vi "_GetBitfiledValue.vi"(8 "error in":errorcluster, 10 "bitfield caps":T1={"offset"=0, "size"=0, "signed?"=TRUE}, 11 "register value":u64=9199446298756579247 format="%.0x") -> (0 "error out":errorcluster, 3 "bitfield balue":variant)   [LabVIEW 2017, in "Bitfield.lvlib"]
uses:
  Bitfield.lvlib
  BitfieldCaps.ctl
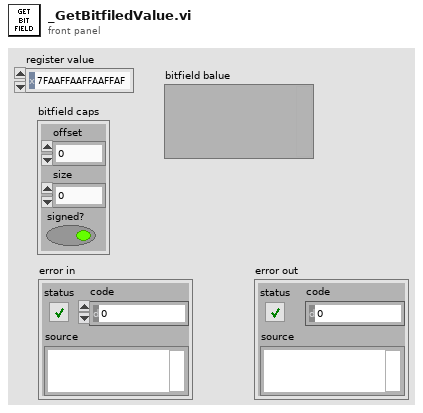
[diagram p1: front panel]
types:
  T1 = typedef "Bitfield.lvlib/BitfieldCaps.ctl" = cluster{"offset":i32, "size":i32, "signed?":bool}
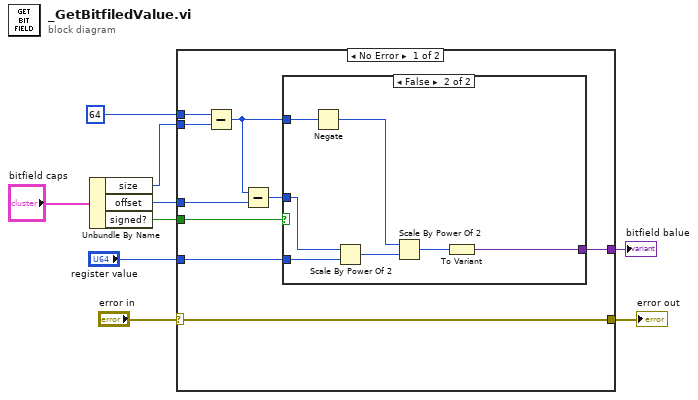
[diagram p0: block diagram]
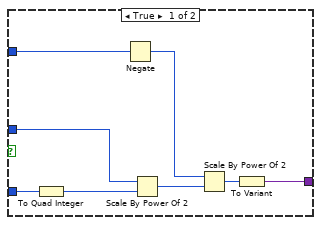
[diagram p2: hidden frame]
diagram:
  n1 = Unbundle By Name("bitfield caps") -> ("size"=w5:i32, "offset"=w4:i32, "signed?"=w3:bool)
  n2 = case shown="No Error" "error in" {
    selector: "error in" -> [w10 w34]
    tunnel: "register value" -> [w18 _]
    tunnel: [w17 _] -> w7
    tunnel: 64 ("length 2") -> [w16 _]
    tunnel: w5 -> [w13 _]
    tunnel: w4 -> [w12 _]
    tunnel: w3 -> [w11 _]
    tunnel: [w10 w34] -> w1
    frame No Error {
      n3 = Subtract(x=w16, y=w13) -> (x-y=w14:i32)
      n4 = Subtract(x=w14, y=w12) -> (x-y=w15:i32)
      n5 = case shown="False" w11 {
        tunnel: w18 -> [w26 w30]
        tunnel: w15 -> [w19 w27]
        tunnel: [w21 w29] -> w17
        tunnel: w14 -> [w20 w28]
        frame True {
          n6 = To Quad Integer(1:w26) -> (0:w22:i64)
          n7 = Negate(x=w20) -> (-x=w23:i32)
          n8 = Scale By Power Of 2(n=w19, x=w22) -> (x*2^n=w25:i64)
          n9 = Scale By Power Of 2(n=w23, x=w25) -> (x*2^n=w24:i64)
          n10 = To Variant(anything=w24) -> (Variant=w21:variant)
        }
        frame False {
          n11 = Negate(x=w28) -> (-x=w31:i32)
          n12 = Scale By Power Of 2(n=w27, x=w30) -> (x*2^n=w33:u64)
          n13 = Scale By Power Of 2(n=w31, x=w33) -> (x*2^n=w32:u64)
          n14 = To Variant(anything=w32) -> (Variant=w29:variant)
        }
      }
    }
    frame Error {
    }
  }
  "bitfield balue" <- w7
  "error out" <- w1
